vi "1A Helper - Init Sensor.vi"(8 "error in (no error)":errorcluster, 11 "VISA Refnum in":refnum<visa-resource-name>="COM1") -> (0 "error out":errorcluster, 2 "Try #":i32, 3 "VISA Refnum out":refnum<visa-resource-name>)   [LabVIEW 2011]
doc: "This VI checks to see if the sensor is communicating on 4800 or 38400 baud and sets it to 38400 baud if it is not already."
uses:
  2-Think/2 Typedefs/indicator LED.ctl
  2-Think/2 Globals/2 Global.vi
panel:
  out "# of serial connection attempts":i32
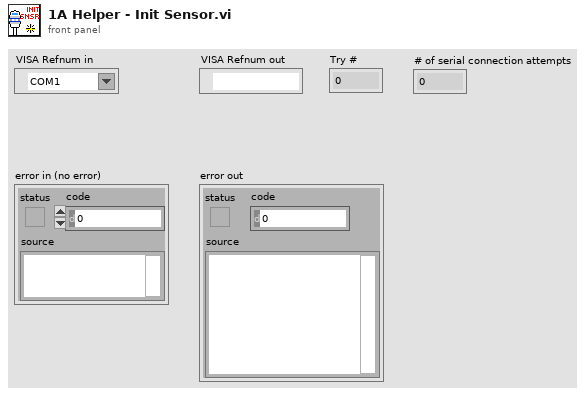
[diagram p1: front panel]
types:
  T1 = typedef "indicator LED.ctl" = bool
  T2 = typedef "generalized sensor status.ctl" = cluster{"Sensor Connected":T1, "Sensor Initialized":T1, "Sensor OK":T1, "Latest Error String":string, "GPS Lock":T1}
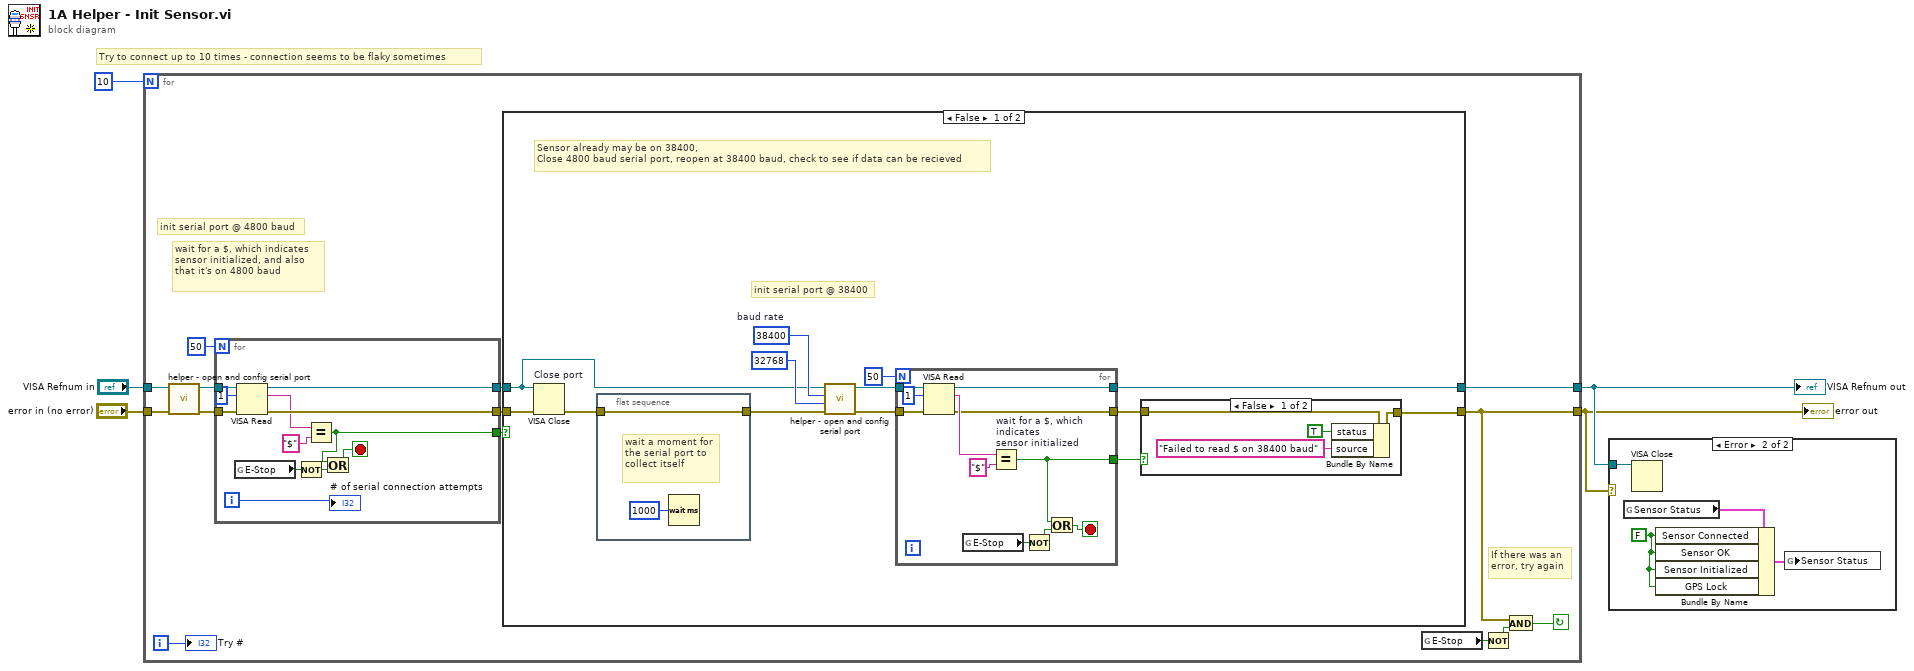
[diagram p0: block diagram]
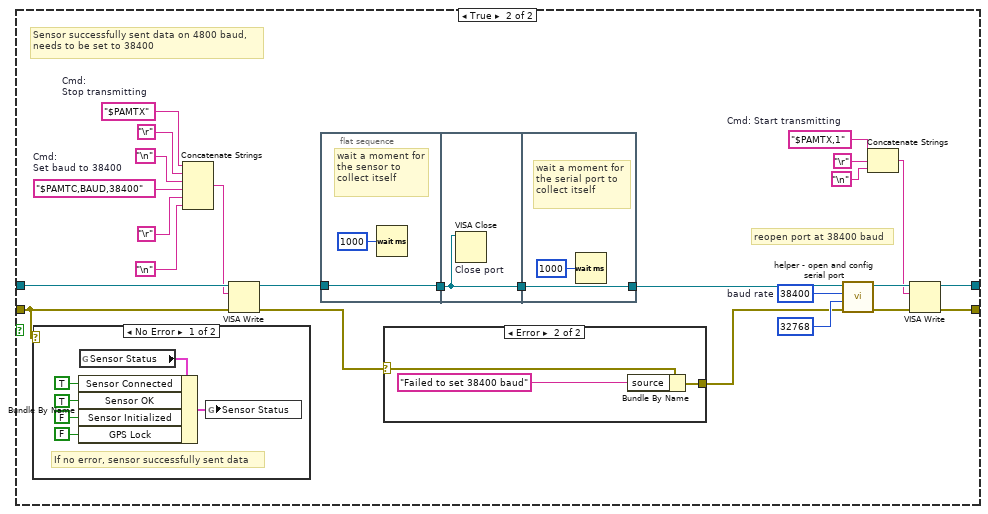
[diagram p3: hidden frame]
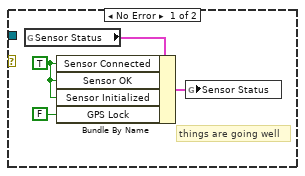
[diagram p6: hidden frame]
diagram:
  # "Try to connect up to 10 times - connection seems to be flaky sometimes"
  n1 = for {
    N: 10 -> [_]
    tunnel: "error in (no error)" -> [w19]
    tunnel: "VISA Refnum in" -> [w18]
    tunnel: [w17] -> w3
    tunnel: [w9] -> w2
    i -> [w11]
    stop <- w10 continue-if-true
    # "If there was an \nerror, try again"
    # "wait for a $, which indicates sensor initialized, and also that it's on 4800 baud"
    # "init serial port @ 4800 baud"
    n2 = call "helper - open and config serial port.vi"("error in (no error)"=w19, "VISA Refnum in"=w18) -> ("error out"=w14:errorcluster, "VISA Refnum out"=w15:refnum<visa-resource-name>)  [unwired: 8 in]
    n3 = for {
      N: 50 -> [_]
      tunnel: [w31] -> w16
      tunnel: w15 -> [w30]
      tunnel: w14 -> [w29]
      tunnel: [w28] -> w13
      tunnel: [w21] -> w12
      i -> [w20]
      stop <- w22 stop-if-true
      n4 = global read "2 Global.vi" "E-Stop"() -> (w23:bool)
      n5 = VISA Read(VISA resource name=w30, byte count=u32 1, error in (no error)=w29) -> (VISA resource name out=w31:refnum<visa-resource-name>, read buffer=w26:string, error out=w28:errorcluster)  [unwired: 1 out]
      n6 = Not(x=w23) -> (.not. x?=w24:bool)
      n7 = Equal? ("wait for a $, which indicates\nsensor initialized")(x=w26, y="$" ("x")) -> (x = y?=w21:bool)
      n8 = Or(x=w21, y=w24) -> (x .or. y?=w22:bool)
      "# of serial connection attempts" <- w20
    }
    n9 = case shown="False" w12 {
      tunnel: [w40 w83] -> w17
      tunnel: w16 -> [w32 w75]
      tunnel: w13 -> [w35 w65]
      tunnel: [w39 w70] -> w9
      frame False {
        w44 = u32 38400  # baud rate
        # "init serial port @ 38400"
        # "Sensor already may be on 38400,\nClose 4800 baud serial port, reopen at 38400 baud, check to see if data can be recieved"
        n10 = VISA Close "Close port"(VISA resource name=w32, error in (no error)=w35) -> (error out=w34:errorcluster)
        n11 = flat-sequence {
          tunnel: w34 -> [w45]
          tunnel: [w45] -> w33
          frame #0 {
            # "wait a moment for the serial port to collect itself"
            n12 = Wait (ms)(milliseconds to wait=u32 1000) -> ()  [unwired: 1 out]
          }
        }
        n13 = call "helper - open and config serial port.vi"("error in (no error)"=w33, "Input\nbuffer size"=u32 32768 ("Input\nbuffer size"), "baud rate"=w44, "VISA Refnum in"=w32) -> ("error out"=w41:errorcluster, "VISA Refnum out"=w42:refnum<visa-resource-name>)  [unwired: 6 in]
        n14 = for {
          N: 50 -> [_]
          tunnel: w42 -> [w57]
          tunnel: w41 -> [w56]
          tunnel: [w55] -> w40
          tunnel: [w47] -> w38
          tunnel: [w51] -> w37
          stop <- w48 stop-if-true
          n15 = VISA Read(VISA resource name=w57, byte count=u32 1, error in (no error)=w56) -> (VISA resource name out=w55:refnum<visa-resource-name>, read buffer=w53:string, error out=w51:errorcluster)  [unwired: 1 out]
          n16 = global read "2 Global.vi" "E-Stop"() -> (w49:bool)
          n17 = Equal? "wait for a $, which indicates\nsensor initialized"(x=w53, y="$" ("x")) -> (x = y?=w47:bool)
          n18 = Not(x=w49) -> (.not. x?=w50:bool)
          n19 = Or(x=w47, y=w50) -> (x .or. y?=w48:bool)
        }
        n20 = case shown="False" w38 {
          tunnel: w37 -> [w59 w62]
          tunnel: [w58 w62] -> w39
          frame False {
            n21 = Bundle By Name(cluster=w59, "status"=TRUE, "source"="Failed to read $ on 38400 baud") -> (w58:errorcluster)
          }
          frame True {
          }
        }
      }
      frame True {
        w69 = "$PAMTC,BAUD,38400"  # Cmd: Set baud to 38400
        w74 = "$PAMTX"  # Cmd: Stop transmitting
        w79 = "$PAMTX,1"  # Cmd: Start transmitting
        w85 = u32 38400  # baud rate
        # "Sensor successfully sent data on 4800 baud,\nneeds to be set to 38400"
        # "reopen port at 38400 baud"
        n22 = case shown="No Error" w65 {
          frame No Error {
            # "If no error, sensor successfully sent data"
            n23 = global read "2 Global.vi" "Sensor Status"() -> (w96:T2)
            n24 = Bundle By Name(cluster=w96, "Sensor Connected"=T1 TRUE, "Sensor OK"=T1 TRUE, "Sensor Initialized"=T1 FALSE, "GPS Lock"=T1 FALSE) -> (w97:T2)
            n25 = global write "2 Global.vi" "Sensor Status"(w97) -> ()
          }
          frame Error {
          }
        }
        n26 = Concatenate Strings(w74, "\r" ("Carriage Return Constant"), "\n", w69, "\r" ("Carriage Return Constant"), "\n") -> (w73:string)
        n27 = VISA Write(VISA resource name=w75, write buffer=w73, error in (no error)=w65) -> (VISA resource name out=w66:refnum<visa-resource-name>, error out=w64:errorcluster)  [unwired: 1 out]
        n28 = flat-sequence {
          tunnel: w66 -> [w98]
          tunnel: [w98] -> w87
          tunnel: w87 -> [w100]
          tunnel: [w100] -> w86
          tunnel: [w102] -> w84
          tunnel: w86 -> [w102]
          frame #0 {
            # "wait a moment for the sensor to collect itself"
            n29 = Wait (ms)(milliseconds to wait=u32 1000) -> ()  [unwired: 1 out]
          }
          frame #1 {
            n30 = VISA Close "Close port"(VISA resource name=w100) -> ()  [unwired: 1 in, 1 out]
          }
          frame #2 {
            # "wait a moment for the serial port to collect itself"
            n31 = Wait (ms)(milliseconds to wait=u32 1000) -> ()  [unwired: 1 out]
          }
        }
        n32 = case shown="Error" w64 {
          selector: w64 -> [w88 w91]
          tunnel: [w88 w89] -> w63
          frame No Error {
          }
          frame Error {
            n33 = Bundle By Name(cluster=w91, "source"="Failed to set 38400 baud") -> (w89:errorcluster)
          }
        }
        n34 = call "helper - open and config serial port.vi"("error in (no error)"=w63, "Input\nbuffer size"=u32 32768 ("Input\nbuffer size"), "baud rate"=w85, "VISA Refnum in"=w84) -> ("error out"=w82:errorcluster, "VISA Refnum out"=w80:refnum<visa-resource-name>)  [unwired: 6 in]
        n35 = Concatenate Strings(w79, "\r" ("Carriage Return Constant"), "\n") -> (w76:string)
        n36 = VISA Write(VISA resource name=w80, write buffer=w76, error in (no error)=w82) -> (VISA resource name out=w83:refnum<visa-resource-name>, error out=w70:errorcluster)  [unwired: 1 out]
      }
    }
    n37 = global read "2 Global.vi" "E-Stop"() -> (w7:bool)
    n38 = Not(x=w7) -> (.not. x?=w8:bool)
    n39 = And(x=w9, y=w8) -> (x .and. y?=w10:bool)
    "Try #" <- w11
  }
  "VISA Refnum out" <- w3
  "error out" <- w2
  n40 = case shown="Error" w2 {
    tunnel: w3 -> [_ w110]
    frame No Error {
      w104 = T1 TRUE ("Sensor Connected")
      # "things are going well"
      n41 = global read "2 Global.vi" "Sensor Status"() -> (w105:T2)
      n42 = Bundle By Name(cluster=w105, "Sensor Connected"=w104, "Sensor OK"=w104, "Sensor Initialized"=w104, "GPS Lock"=T1 FALSE) -> (w106:T2)
      n43 = global write "2 Global.vi" "Sensor Status"(w106) -> ()
    }
    frame Error {
      w107 = T1 FALSE ("Sensor Connected")
      n44 = global read "2 Global.vi" "Sensor Status"() -> (w108:T2)
      n45 = VISA Close(VISA resource name=w110) -> ()  [unwired: 1 in, 1 out]
      n46 = Bundle By Name(cluster=w108, "Sensor Connected"=w107, "Sensor OK"=w107, "Sensor Initialized"=w107, "GPS Lock"=w107) -> (w109:T2)
      n47 = global write "2 Global.vi" "Sensor Status"(w109) -> ()
    }
  }
